vi "Calculate FPGA Loop Rate.vi"(10 "FPGA Clock Freq":u32=40000000, 11 "Loop Frequency (Hz)":dbl=1000000.0) -> (3 "Loop  Rate (ticks)":u32)   [LabVIEW 2017]
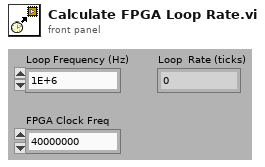
[diagram p1: front panel]
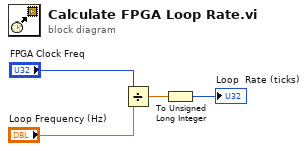
[diagram p0: block diagram]
diagram:
  n1 = Divide(x="FPGA Clock Freq", y="Loop Frequency (Hz)") -> (x/y=w3:dbl)
  n2 = To Unsigned Long Integer(number=w3) -> (unsigned 32bit integer=→"Loop  Rate (ticks)":u32)
